vi "Position other mission menu Button.vi"(8 "error in (no error)":errorcluster, 10 "Previous Button":refnum<vi>, 11 "Button Ref":refnum<vi>) -> (0 "error out":errorcluster)   [LabVIEW 2014]
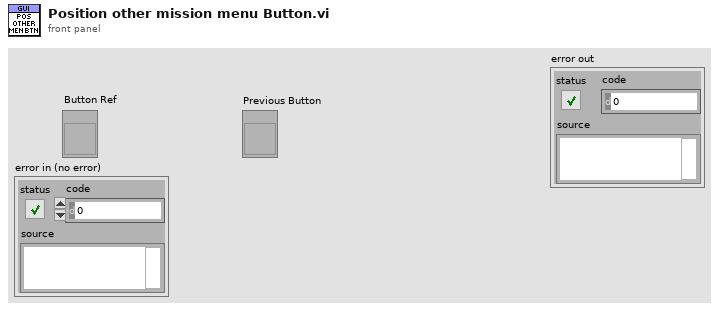
[diagram p1: front panel]
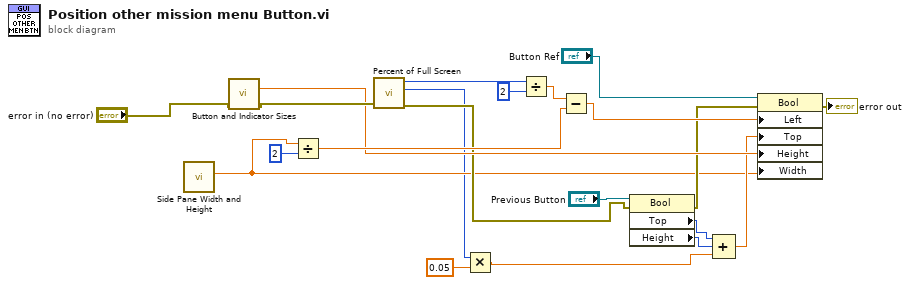
[diagram p0: block diagram]
diagram:
  n1 = call "Side Pane Width and Height.vi"() -> ("Width"=w4:dbl)  [unwired: 9 in, 2 out]
  n2 = call "Button and Indicator Sizes.vi"("error in (no error)"="error in (no error)") -> ("Button Height"=w11:dbl, "error out"=w13:errorcluster)  [unwired: 10 in, 3 out]
  n3 = Divide(x=w4, y=u32 2) -> (x/y=w17:dbl)
  n4 = call "Percent of Full Screen.vi"("error in (no error)"=w13) -> ("error out"=w9:errorcluster, "Bottom"=w3:i16, "Right"=w20:i16)  [unwired: 8 in]
  n5 = Multiply(x=w3, y=0.05) -> (x*y=w1:dbl)
  n6 = Divide(x=w20, y=i16 2) -> (x/y=w18:dbl)
  n7 = Subtract(x=w18, y=w17) -> (x-y=w16:dbl)
  n8 = property class="Bool"(reference="Previous Button", error in=w9) -> (error out=w8:errorcluster, "Top"=w7:i32, "Height"=w6:u32)  [unwired: 1 out]
  n9 = Compound Arithmetic op=ADD(w7, w6, w1) -> (w5:dbl)
  n10 = property class="Bool"(reference="Button Ref", error in=w8, "Left"=w16, "Top"=w5, "Height"=w11, "Width"=w4) -> (error out=→"error out":errorcluster)  [unwired: 1 out]
